vi "Get Pattern Data.vi"(9 "File Name":i32[](array[numeric]), 10 "Folder Name":string, 11 "Dispense.lvclass":refnum<class "Dispense.lvclass">) -> (3 "Dispense Out":refnum<class "Dispense.lvclass">)   [LabVIEW 2020, in "Dispense.lvclass"]
uses:
  Dispense.lvclass
  Dispense.lvclass/Dispense.ctl
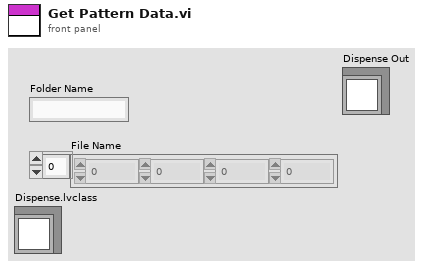
[diagram p1: front panel]
types:
  T1 = typedef "File Paths.ctl" = cluster{"Glue Pattern Folder":path, "Carrier Tray Folder":path, "Pick Up Tool Fixture Folder":path, "Components Folder":path, "Bellows Tool Offset.txt":path, "Pick Up Tool Offset.txt":path, "Dispense Tip Offset.txt":path, "Log Files":path}
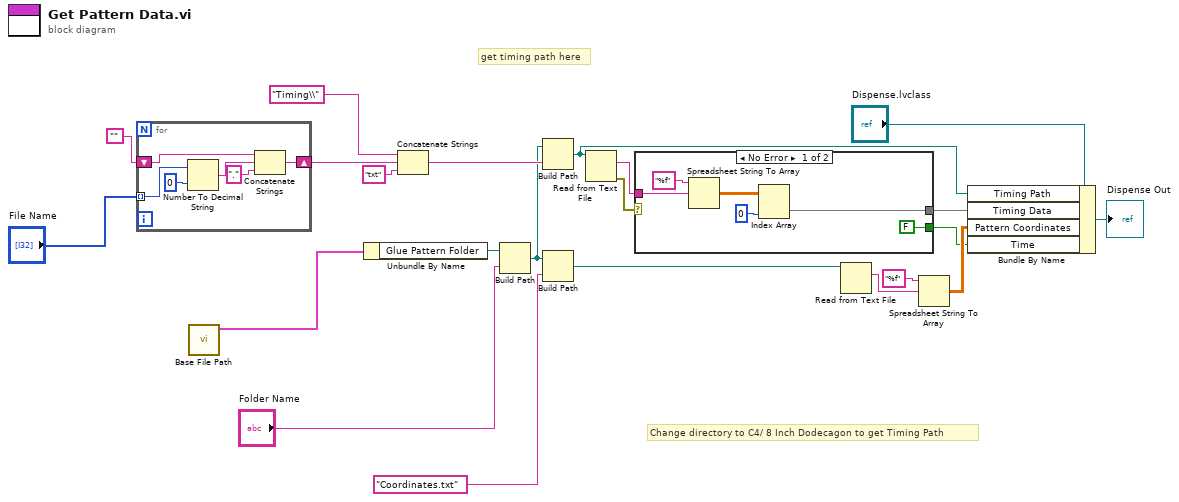
[diagram p0: block diagram]
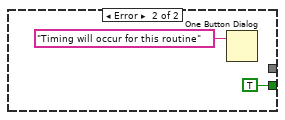
[diagram p2: hidden frame]
diagram:
  # "Change directory to C4/ 8 Inch Dodecagon to get Timing Path"
  # "get timing path here"
  n1 = for {
    tunnel: "File Name" -> [w28] mode=indexing
    shift-right: [w24] -> w18
    shift-left: "" -> [w23]
    n2 = Number To Decimal String(number=w28, width (-)=i16 0) -> (decimal integer string=w26:string)
    n3 = Concatenate Strings(w23, w26, "." ("string")) -> (w24:string)
  }
  n4 = call "Base File Path.vi"() -> ("Paths Out"=w9:T1)  [unwired: 11 in]
  n5 = Unbundle By Name(w9) -> ("Glue Pattern Folder"=w13:path)
  n6 = Concatenate Strings("Timing\\" ("name or relative path"), w18, "txt" ("string")) -> (w21:string)
  n7 = Build Path(base path=w13, name or relative path="Folder Name") -> (appended path=w20:path)
  n8 = Build Path(base path=w20, name or relative path=w21) -> (appended path=w7:path)
  n9 = Build Path(base path=w20, name or relative path="Coordinates.txt") -> (appended path=w15:path)
  n10 = Read from Text File(file (use dialog)=w7) -> (text=w22:string, error out=w1:errorcluster)  [unwired: 3 in, 2 out]
  n11 = case shown="No Error" w1 {
    tunnel: w22 -> [w33 _]
    tunnel: [w31 _] -> w6
    tunnel: [FALSE TRUE] -> w4
    frame No Error {
      n12 = Spreadsheet String To Array(format string="%f", spreadsheet string=w33) -> (array=w32:dbl[][])  [unwired: 2 in]
      n13 = Index Array(array=w32, index (col)=0 ("disabled index (col)")) -> (element=w31:dbl[])  [unwired: 1 in]
    }
    frame Error {
      n14 = One Button Dialog(message="Timing will occur for this routine") -> ()  [unwired: 1 in, 1 out]
    }
  }
  n15 = Read from Text File(file (use dialog)=w15) -> (text=w11:string)  [unwired: 3 in, 3 out]
  n16 = Spreadsheet String To Array(format string="%f", spreadsheet string=w11) -> (array=w5:dbl[][])  [unwired: 2 in]
  n17 = Bundle By Name(cluster="Dispense.lvclass", "Timing Path"=w7, "Timing Data"=w6, "Pattern Coordinates"=w5, "Time"=w4) -> (→"Dispense Out":refnum<class "Dispense.lvclass">)
